vi "Test TDMS store recall.vi"() -> ()   [LabVIEW 2016]
uses:
  <vilib>/Utility/Data Type/Type Definitions/Data Type.ctl
  <vilib>/Utility/Data Type/Type Definitions/Type Definition Info.ctl
  <vilib>/Utility/Data Type/NI_Data Type.lvlib
panel:
  out "Value out":variant
  out "Parameter out":timestamp
  in  "File Path Control":path=path "C:/Data/test.tdms"
  out "Type Definition Info":T1
  out "Type Definition":bool
  out "Name":string
  out "Type":T2
  in  "Parameter":cluster{"Numeric Control":dbl, "Boolean":bool}
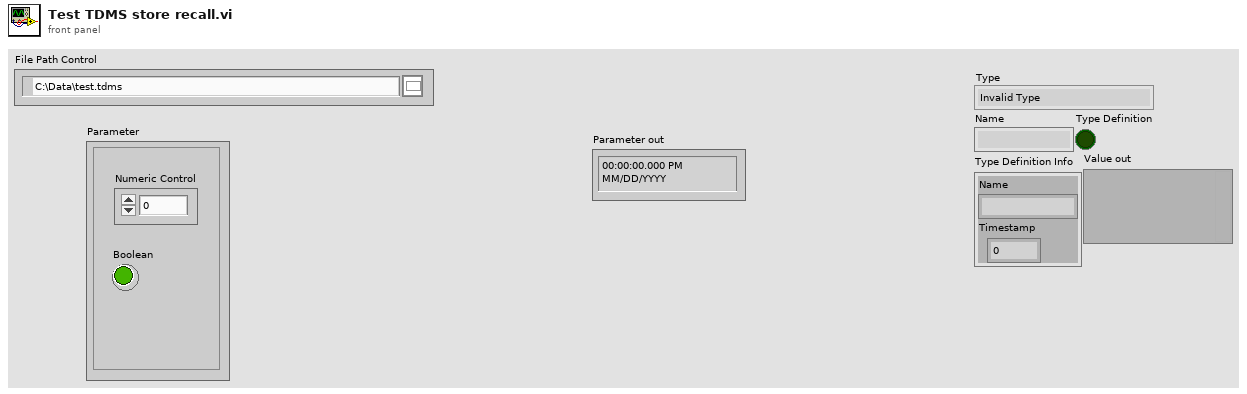
[diagram p1: front panel]
types:
  T1 = typedef "NI_Data Type.lvlib/Type Definition Info.ctl" = cluster{"Name":string, "Timestamp":u32}
  T2 = typedef "NI_Data Type.lvlib/Data Type.ctl" = enum8{"Invalid Type", "Void", "I8", "I16", "I32", "I64", "U8", "U16", "U32", "U64", "Single Float", "Double Float", "Extended Float", "Single Complex", "Double Complex", "Extended Complex", "Enum U8", "Enum U16", "Enum U32", "Enum U64", "Single Float With Unit", "Double Float With Unit", "Extended Float With Unit", "Single Complex with Unit", "Double Complex with Unit", "Extended Complex with Unit", "Boolean", "String", "Path", "Picture", "Tag", "Array", "Cluster", "Variant", "LV Variant", "Waveform", "Timestamp", "Digital Waveform", "Digital Data", "ExpressData", "Refnum", "External Data", "VI", "Poly VI", "LabVIEW Class Instance", "Fixed Point"}
  T3 = enum16{"open", "open or create", "create or replace", "create", "open (read-only)"}
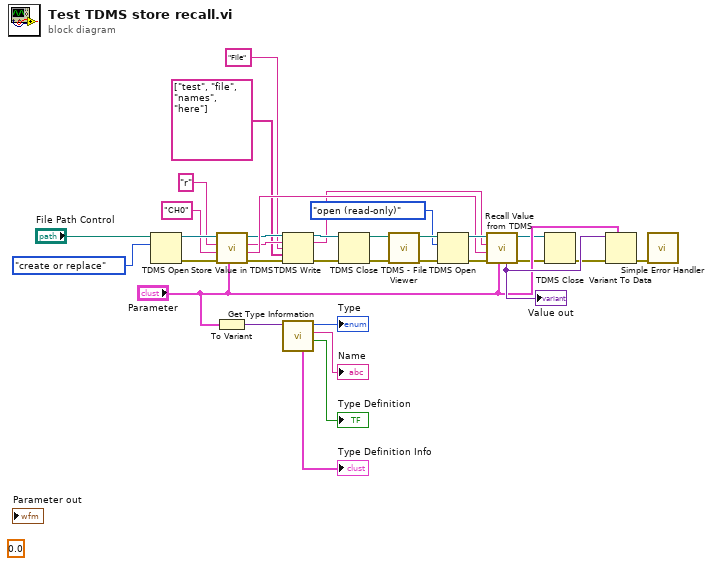
[diagram p0: block diagram]
diagram:
  (unwired) 0.0 ("Numeric Control")
  n1 = TDMS Open(10:T3."create or replace" ("operation (0:open)"), 11:"File Path Control") -> (0:w25:errorcluster, 3:w27:refnum<k34>)  [unwired: 5 in]
  n2 = call "Store Value in TDMS.vi"("Value"="Parameter", "Error In"=w25, "channel name"="CH0", "group name"="r", "tdms file"=w27) -> ("Error Out"=w4:errorcluster, "channel name out"=w10:string, "group name out"=w6:string, "tdms file out"=w8:refnum<k34>)  [unwired: 3 in]
  n3 = To Variant(anything="Parameter") -> (Variant=w33:variant)
  n4 = TDMS Write(0:w8, 5:w6, 7:"File", 9:string[] ["test", "file", "names", "here"], 11:w4) -> (4:w7:refnum<k34>, 6:w5:string, 15:w3:errorcluster)  [unwired: 1 in, 1 out]
  n5 = call <vilib>:"Get Type Information.vi"("Variant"=w33) -> ("Type Definition"=→"Type Definition":bool, "Name"=→"Name":string, "Type"=→"Type":T2, "Type Definition Info"=→"Type Definition Info":T1)  [unwired: 6 in, 1 out]
  n6 = TDMS Close(8:w3, 11:w7) -> (0:w22:errorcluster, 3:w21:path)
  n7 = call <vilib>:"TDMS - File Viewer.vi"("error in (no error)"=w22, "file path"=w21) -> ("error out"=w19:errorcluster, "file path out"=w18:path)  [unwired: 4 in]
  n8 = TDMS Open(8:w19, 10:T3."open (read-only)" ("operation (0:open)"), 11:w18) -> (0:w11:errorcluster, 3:w15:refnum<k34>)  [unwired: 4 in]
  n9 = call "Recall Value from TDMS.vi"("Value"="Parameter", "Error In"=w11, "channel name"=w10, "group name"=w5, "tdms file"=w15) -> ("Error Out"=w14:errorcluster, "tdms file out"=w12:refnum<k34>, "Value out"=w20:variant)  [unwired: 2 in, 2 out]
  "Value out" <- w20
  n10 = TDMS Close(8:w14, 11:w12) -> (0:w13:errorcluster)  [unwired: 1 out]
  n11 = Variant To Data(error in=w13, type="Parameter", Variant=w20) -> (error out=w9:errorcluster)  [unwired: 1 out]
  n12 = call <vilib>:"Simple Error Handler.vi"("error in (no error)"=w9) -> ()  [unwired: 4 in, 5 out]
